vi "游戏初始化.vi"(10 "列数":dbl, 11 "行数":dbl) -> (2 "雷区":dbl[][](array[numeric]), 3 "地图":dbl[][](array[numeric]))   [LabVIEW 2012]
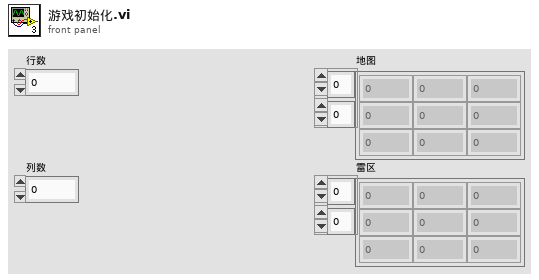
[diagram p1: front panel]
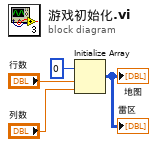
[diagram p0: block diagram]
diagram:
  n1 = Initialize Array(0, "行数", "列数") -> (→"地图" →"雷区":i32[][])
